vi "Recieve command.vi"(0 "reference in":refnum<class "ZMQ_slave.lvclass">, 11 "error in (no error)":errorcluster, 13 "timeout ms (100)":i32=100) -> (4 "reference out":refnum<class "ZMQ_slave.lvclass">, 6 "message":string, 8 "parameters":string, 10 "data":variant, 14 "timed out?":bool, 15 "error out":errorcluster)   [LabVIEW 2019, in "CommandResponse communication.lvlib" / "ZMQ_slave.lvclass"]
doc: "Recives command as message + variant data"
uses:
  ZMQ_slave.lvclass
  <vilib>/addons/zeromq/zmq_socket.lvclass
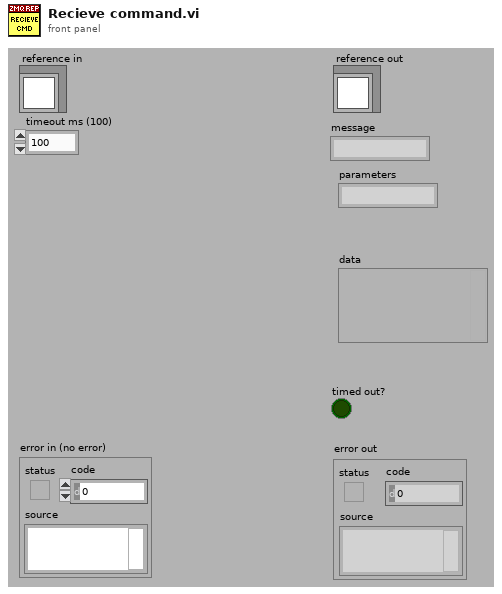
[diagram p1: front panel]
types:
  T1 = enum16{"big-endian, network order", "native, host order", "little-endian"}
  T2 = typedef "CommandResponse communication.lvlib/ZMQ_slave.lvclass/ObjectAttributes.ctl" = cluster{"ZMQ context":refnum<class "zmq_context.lvclass">, "ZMQ socket":refnum<class "zmq_socket.lvclass">, "endpoint":string}
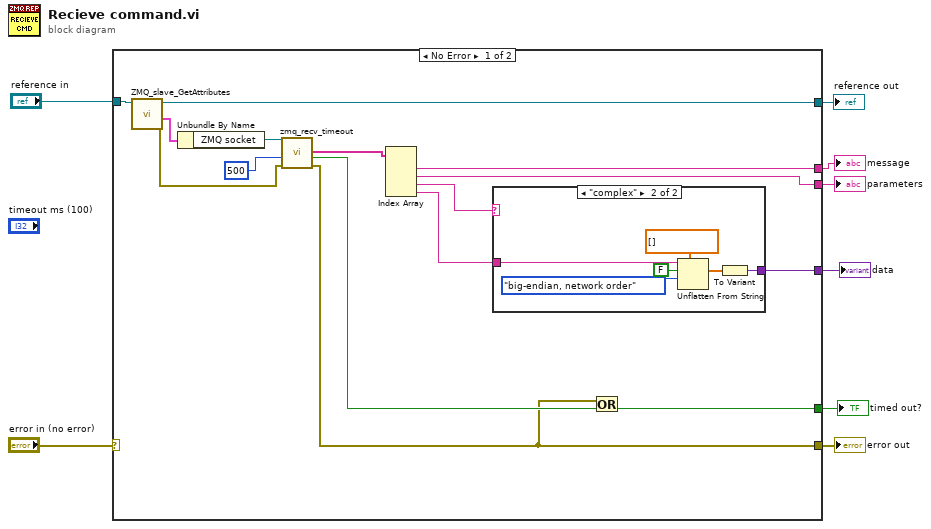
[diagram p0: block diagram]
diagram:
  n1 = case shown="No Error" "error in (no error)" {
    selector: "error in (no error)" -> [_ w31]
    tunnel: [w10 w31] -> w7
    tunnel: [w23 w30] -> w5
    tunnel: "reference in" -> [w21 w30]
    tunnel: [w18 _] -> w4
    tunnel: [w17 _] -> w3
    tunnel: [w13 _] -> w2
    tunnel: [w11 _] -> w1
    frame No Error {
      n2 = call "ZMQ_slave_GetAttributes.vi"("reference in"=w21) -> ("error out"=w14:errorcluster, "attributes"=w22:T2, "reference out"=w23:refnum<class "ZMQ_slave.lvclass">)  [unwired: 7 in, 1 out]
      n3 = Unbundle By Name(w22) -> ("ZMQ socket"=w20:refnum<class "zmq_socket.lvclass">)
      n4 = call <vilib>:"zmq_recv_timeout.vi"("error in"=w14, "timeout (ms)"=u32 500, "socket in"=w20) -> ("error out"=w10:errorcluster, "timeout?"=w12:bool, "parts"=w9:string[])  [unwired: 1 in, 1 out]
      n5 = Index Array(array=w9) -> (element #1=w18:string, element #2=w17:string, element #3=w16:string, element #4=w15:string)  [unwired: 4 in]
      n6 = case shown="\"complex\"" w16 {
        tunnel: w15 -> [_ w29]
        tunnel: [_ w24] -> w13
        frame "False", Default {
        }
        frame "complex" {
          n7 = Unflatten From String(type=csg[] [], binary string=w29, data includes array or string size? (T)=FALSE, byte order (0:big-endian, network order)=T1."big-endian, network order") -> (value=w25:csg[])  [unwired: 1 in, 2 out]
          n8 = To Variant(anything=w25) -> (Variant=w24:variant)
        }
      }
      n9 = Or(x=w10, y=w12) -> (x .or. y?=w11:bool)
    }
    frame Error {
    }
  }
  "error out" <- w7
  "reference out" <- w5
  "message" <- w4
  "parameters" <- w3
  "data" <- w2
  "timed out?" <- w1
